vi "Get Profile.vi"(8 "error in (no error)":errorcluster, 11 "MotorDrive in":refnum<class "MotorDrive.lvclass">) -> (0 "error out":errorcluster, 1 "Setpoint Deceleration":u32, 2 "Setpoint Acceleration":u32, 3 "MotorDrive out":refnum<class "MotorDrive.lvclass">, 4 "Setpoint Position":i32, 5 "Setpoint Velocity":u32)   [LabVIEW 2016, in "MotorDrive.lvclass"]
uses:
  MotorDrive.lvclass
  MotorDrive.lvclass/MotorDrive.ctl
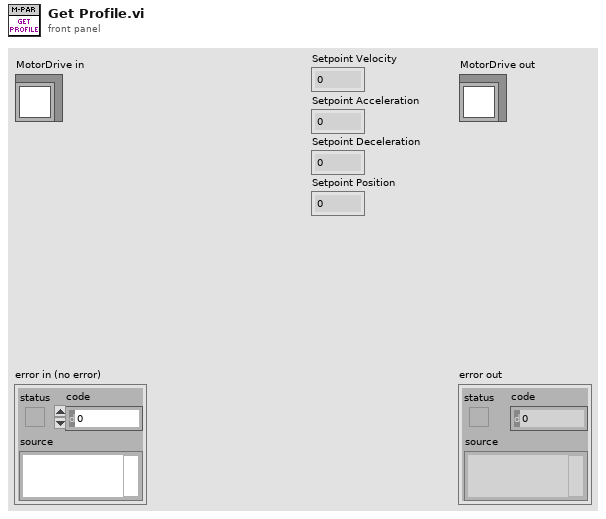
[diagram p1: front panel]
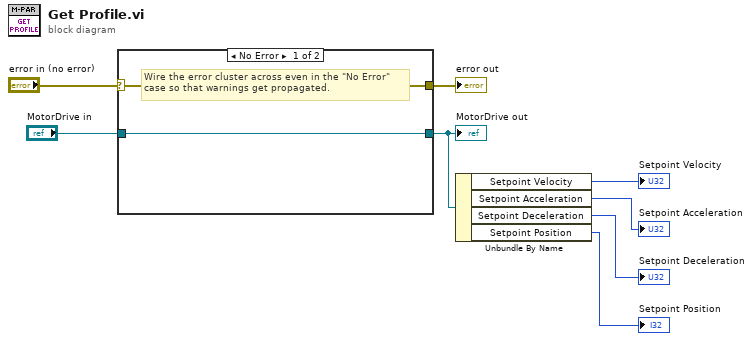
[diagram p0: block diagram]
diagram:
  n1 = case shown="No Error" "error in (no error)" {
    selector: "error in (no error)" -> [w10 w12]
    tunnel: [w10 w12] -> w7
    tunnel: [w9 w11] -> w5
    tunnel: "MotorDrive in" -> [w9 w11]
    frame No Error {
      # "Wire the error cluster across even in the \"No Error\"\ncase so that warnings get propagated."
    }
    frame Error {
    }
  }
  "error out" <- w7
  "MotorDrive out" <- w5
  n2 = Unbundle By Name(w5) -> ("Setpoint Velocity"=→"Setpoint Velocity":u32, "Setpoint Acceleration"=→"Setpoint Acceleration":u32, "Setpoint Deceleration"=→"Setpoint Deceleration":u32, "Setpoint Position"=→"Setpoint Position":i32)
